vi "pasos a mover.vi"(11 "Datos de Nueva Adquisición In":T1={"Montura"=enum."Motor Bipolar", "Equipo a Utilizar"=enum."TDS 2012B Osciloscope", "Datos Zaber"={"Sentido de Adquisición"=FALSE, "Comenzar Desde Home?"=FALSE, "Distancia a recorrer (cm)"=0, "Pasos motor"=0, "Distancia entre Lecturas (um)"=0.0, "Puerto"=""}, "Datos Bipolar/Unipolar"={"Puerto COM"="", "Pasos entre Lecturas"=0, "Numero de lecturas"=0, "Sentido del motor"=TRUE}, "Datos Archivo"={"Ruta Archivo"=path "", "Nombre de Prueba"=""}, "Datos actuales"={"Montura"="", "Equipo"="", "Posición Actual"="", "Distancia Total a recorrer"="", "distancia Entre lecturas"="", "Pasos entre lecturas"=""}, "Datos a Guardar In"={"Datos Cursor Tektronix"="", "Datos Lokin"="", "Posición Cero"=0.0, "Posición Actual"=0.0}, "Datos Osciloscopio"={"Sesión Visa Osciloscopio"="Tektronix_TDS2012C", "Tipo de Adquisición"=enum."Voltaje Pico Pico", "Canal a Utilizar"=enum."Canal 1", "Parametros de Adquisición"=enum."Una Muestra", "Número Promedio"=2}, "Datos Lock In"={"Visa Lock in"="Tektronix_TDS2012C"}} {"Datos Osciloscopio"."Número Promedio" min=2 max=20; "Datos a Guardar In"."Posición Actual" format="%#_10f"; "Datos a Guardar In"."Posición Cero" format="%#_10f"; "Datos Bipolar/Unipolar"."Numero de lecturas" max=910098 step=1}) -> (3 "Datos nueva adquisición Out":T1={"Montura"=enum."Motor Bipolar", "Equipo a Utilizar"=enum."TDS 2012B Osciloscope", "Datos Zaber"={"Sentido de Adquisición"=FALSE, "Comenzar Desde Home?"=FALSE, "Distancia a recorrer (cm)"=0, "Pasos motor"=0, "Distancia entre Lecturas (um)"=0.0, "Puerto"=""}, "Datos Bipolar/Unipolar"={"Puerto COM"="", "Pasos entre Lecturas"=0, "Numero de lecturas"=0, "Sentido del motor"=TRUE}, "Datos Archivo"={"Ruta Archivo"=path "", "Nombre de Prueba"=""}, "Datos actuales"={"Montura"="", "Equipo"="", "Posición Actual"="", "Distancia Total a recorrer"="", "distancia Entre lecturas"="", "Pasos entre lecturas"=""}, "Datos a Guardar In"={"Datos Cursor Tektronix"="", "Datos Lokin"="", "Posición Cero"=0.0, "Posición Actual"=0.0}, "Datos Osciloscopio"={"Sesión Visa Osciloscopio"="Tektronix_TDS2012C", "Tipo de Adquisición"=enum."Voltaje Pico Pico", "Canal a Utilizar"=enum."Canal 1", "Parametros de Adquisición"=enum."Una Muestra", "Número Promedio"=2}, "Datos Lock In"={"Visa Lock in"="Tektronix_TDS2012C"}} {"Datos Osciloscopio"."Número Promedio" min=2 max=20; "Datos a Guardar In"."Posición Actual" format="%#_10f"; "Datos a Guardar In"."Posición Cero" format="%#_10f"; "Datos Bipolar/Unipolar"."Numero de lecturas" max=910098 step=1})   [LabVIEW 2020]
doc: "Este Vi realiza la conversion de distancia a pasos dependiendo de la resolución de la montura Zaber"
uses:
  Type Definitions/Asistente de adquisicion Cluster.ctl
  Type Definitions/Datos a Guardar.ctl
  Type Definitions/datos osciloscopio.ctl
  Type Definitions/Datos Zaber.ctl
  Type Definitions/parametros motores.ctl
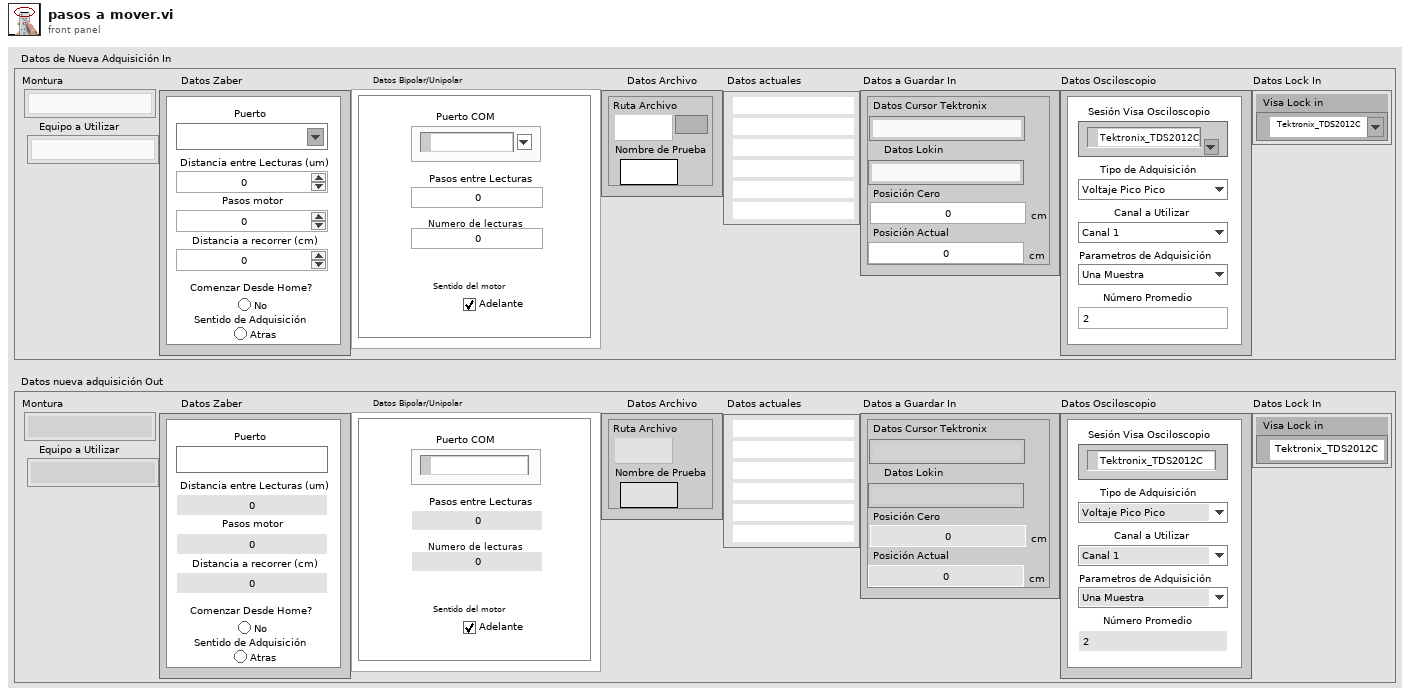
[diagram p1: front panel]
types:
  T1 = typedef "Asistente de adquisicion Cluster.ctl" = cluster{"Montura":enum16{"Zaber T-LSR450B", "Motor Bipolar", "Motor Unipolar"}, "Equipo a Utilizar":enum16{"SR830 Lock In", "TDS 2012B Osciloscope"}, "Datos Zaber":T2, "Datos Bipolar/Unipolar":T3, "Datos Archivo":cluster{"Ruta Archivo":path, "Nombre de Prueba":string}, "Datos actuales":cluster{"Montura":string, "Equipo":string, "Posición Actual":string, "Distancia Total a recorrer":string, "distancia Entre lecturas":string, "Pasos entre lecturas":string}, "Datos a Guardar In":T4, "Datos Osciloscopio":T5, "Datos Lock In":cluster{"Visa Lock in":refnum<visa-resource-name>}}
  T2 = typedef "Datos Zaber.ctl" = cluster{"Sentido de Adquisición":bool, "Comenzar Desde Home?":bool, "Distancia a recorrer (cm)":u32, "Pasos motor":i32, "Distancia entre Lecturas (um)":dbl, "Puerto":refnum<visa-resource-name>}
  T3 = typedef "parametros motores.ctl" = cluster{"Puerto COM":refnum<visa-resource-name>, "Pasos entre Lecturas":u16, "Numero de lecturas":u32, "Sentido del motor":bool}
  T4 = typedef "Datos a Guardar.ctl" = cluster{"Datos Cursor Tektronix":string, "Datos Lokin":string, "Posición Cero":dbl[unit], "Posición Actual":dbl[unit]}
  T5 = typedef "datos osciloscopio.ctl" = cluster{"Sesión Visa Osciloscopio":refnum<visa-resource-name>, "Tipo de Adquisición":enum16{"Voltaje Pico Pico", "Voltaje RMS", "Cursor Tiempo"}, "Canal a Utilizar":enum16{"Canal 1", "Canal 2", "Canal 1 y 2"}, "Parametros de Adquisición":enum16{"Una Muestra", "Promedio"}, "Número Promedio":i32}
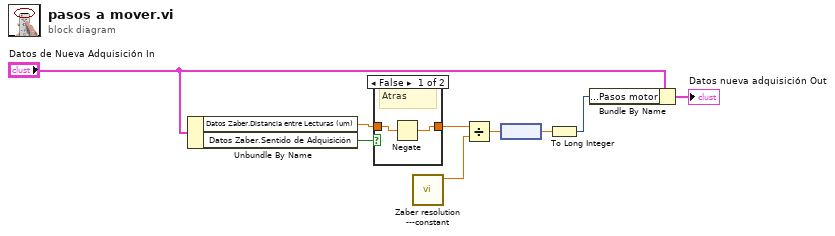
[diagram p0: block diagram]
diagram:
  n1 = Unbundle By Name("Datos de Nueva Adquisición In") -> ("Datos Zaber.Distancia entre Lecturas (um)"=w8:dbl, "Datos Zaber.Sentido de Adquisición"=w9:bool)
  n2 = case shown="False" w9 {
    tunnel: w8 -> [w11 w12]
    tunnel: [w10 w12] -> w7
    frame False {
      # "Atras"
      n3 = Negate(x=w11) -> (-x=w10:dbl)
    }
    frame True {
      # "Adelante"
    }
  }
  n4 = call "Zaber resolution ---constant.vi"() -> ("Resolución"=w6:dbl[unit])  [unwired: 11 in]
  n5 = Divide(x=w7, y=w6) -> (x/y=w5:dbl[unit])
  n6 = node(w5) -> (w4:dbl)
  n7 = To Long Integer(number=w4) -> (32bit integer=w1:i32)
  n8 = Bundle By Name(cluster="Datos de Nueva Adquisición In", "Datos Zaber.Pasos motor"=w1) -> (→"Datos nueva adquisición Out":T1)
